vi "Test_Obtain Message Queue.vi"(8 "error in (no error)":errorcluster, 11 "Queue Name":string) -> (0 "error out":errorcluster, 3 "Message Queue":refnum<queue>)   [LabVIEW 2024, in "Test_2.lvlib" / "Test Message Queue.lvlib"]
doc: "Create a queue with the Message Cluster data type."
uses:
  Test Message Queue.lvlib
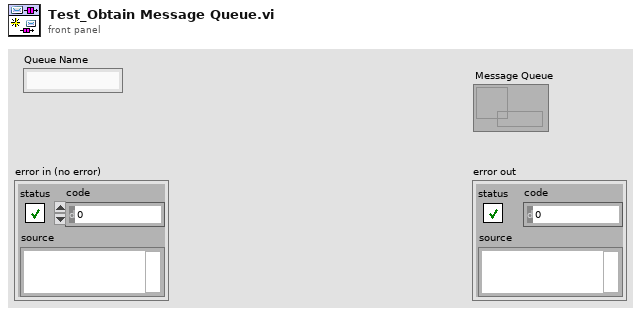
[diagram p1: front panel]
types:
  T1 = cluster{"Message":string, "Message Data":variant}
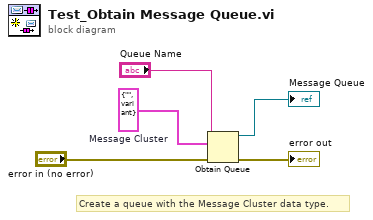
[diagram p0: block diagram]
diagram:
  w5 = T1 {"Message"="", "Message Data"=variant}  # Message Cluster
  # "Create a queue with the Message Cluster data type."
  n1 = Obtain Queue(name (unnamed)="Queue Name", element data type=w5, error in (no error)="error in (no error)") -> (queue out=→"Message Queue":refnum<queue>, error out=→"error out":errorcluster)  [unwired: 2 in, 1 out]
